vi "Core.vi"(8 "error in (no error)":errorcluster, 10 "Actor in":refnum<class "Actor.lvclass">, 11 "Instrument Msg in":refnum<class "Instrument Msg.lvclass">) -> (0 "error out":errorcluster, 1 "Data":refnum<class "Data.lvclass">, 2 "Actor out":refnum<class "Actor.lvclass">, 3 "Instrument Msg out":refnum<class "Instrument Msg.lvclass">)   [LabVIEW 2020, in "Instrument Handler.lvlib" / "Instrument Msg.lvclass"]
doc: "Core of the Reponse Msg. Put the active code here.\n\nThis implementation extract the Instrument from the Instrument Owner and calls Instrument Do Core, where the actual instrument interaction takes place."
uses:
  Instrument Msg.lvclass
  PPL/HDH.Data.Generic.lvlibp/Data.lvclass
  PPL/HDH.Actor Framework.Core.Actor.lvlibp/1abvi3w/vi.lib/ActorFramework/Actor/Actor.lvclass
  Instrument Owner/Instrument Owner.lvclass
  C:/Current projects/WS/PPL/HDH.Actor Framework.Core.Actor.lvlibp/1abvi3w/vi.lib/ActorFramework/Actor/Actor.lvclass
  Instrument Sequencer/Instrument Sequencer.lvclass/Instrument Sequencer.ctl
  Instrument Sequencer/Instrument Sequencer.lvclass
  PPL/HDH.Actor Framework.Core.Instrument Driver.lvlibp/Instrument Driver/Instrument Driver.lvclass
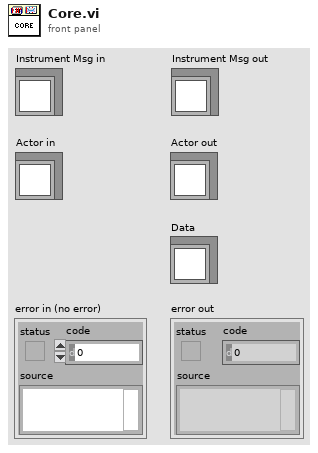
[diagram p1: front panel]
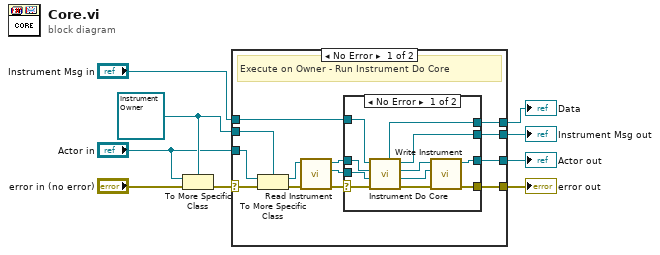
[diagram p0: block diagram]
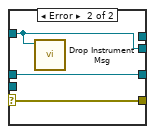
[diagram p2: hidden frame]
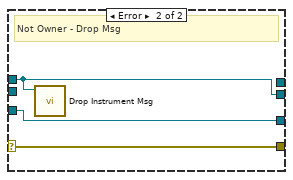
[diagram p3: hidden frame]
diagram:
  w6 = refnum<class "Instrument Owner.lvclass"> refnum ("Instrument Handler.lvlib:Instrument Owner.lvclass")
  n1 = To More Specific Class(target class=w6, reference="Actor in", error in="error in (no error)") -> (error out=w9:errorcluster)  [unwired: 1 out]
  n2 = case shown="No Error" w9 {
    selector: w9 -> [w22 w37]
    tunnel: [w12 w39] -> w8
    tunnel: "Instrument Msg in" -> [w11 w39]
    tunnel: w6 -> [w21 _]
    tunnel: "Actor in" -> [w20 w38]
    tunnel: [w17 w38] -> w4
    tunnel: [w16 w37] -> w3
    tunnel: [w10 _] -> w2
    frame No Error {
      # "Execute on Owner - Run Instrument Do Core"
      n3 = To More Specific Class(target class=w21, reference=w20, error in=w22) -> (specific class reference=w19:refnum<class "Instrument Owner.lvclass">, error out=w18:errorcluster)
      n4 = call "Read Instrument.vi"("error in (no error)"=w18, "Instrument Owner in"=w19) -> ("error out"=w14:errorcluster, "Instrument out"=w13:refnum<class "Instrument Driver.lvclass">, "Instrument Owner out"=w15:refnum<class "Instrument Owner.lvclass">)  [unwired: 7 in]
      n5 = case shown="No Error" w14 {
        selector: w14 -> [w28 w34]
        tunnel: [w33 w36] -> w17
        tunnel: [w32 w34] -> w16
        tunnel: w15 -> [w31 w36]
        tunnel: w13 -> [w30 _]
        tunnel: [w25 w35] -> w12
        tunnel: w11 -> [w26 w35]
        tunnel: [w24 _] -> w10
        frame No Error {
          n6 = call-dynamic "Instrument Do Core.vi"("error in (no error)"=w28, "Instrument in"=w30, "Actor in"=w31, "Instrument Msg in"=w26) -> ("error out"=w27:errorcluster, "Instrument out"=w29:refnum<class "Instrument Driver.lvclass">, "Actor out"=w23:refnum<class "Actor.lvclass">, "Instrument Msg out"=w25:refnum<class "Instrument Msg.lvclass">, "Data"=w24:refnum<class "Data.lvclass">)  [unwired: 3 in]
          n7 = call "Write Instrument.vi"("error in (no error)"=w27, "Instrument in"=w29, "Actor in"=w23) -> ("error out"=w32:errorcluster, "Instrument Owner out"=w33:refnum<class "Instrument Owner.lvclass">)  [unwired: 7 in]
        }
        frame Error {
          n8 = call "Drop Instrument Msg.vi"("Instrument Msg in"=w35) -> ()  [unwired: 11 in]
        }
      }
    }
    frame Error {
      # "Not Owner - Drop Msg"
      n9 = call "Drop Instrument Msg.vi"("Instrument Msg in"=w39) -> ()  [unwired: 11 in]
    }
  }
  "error out" <- w3
  "Actor out" <- w4
  "Data" <- w2
  "Instrument Msg out" <- w8
